vi "DCSMBReadXTemplateJK2.vi"(3 ";error in (no error)":errorcluster, 5 ";Type":i32, 6 ";DataIn 2":string) -> (0 "error IO":errorcluster, 1 "Time Stamp":timestamp, 2 ";DataIn":string)   [LabVIEW 2017]
uses:
  <vilib>/variable/detnetvar/DSV init parameters.ctl
  <vilib>/variable/detnetvar/Network provider/lvedc.dll
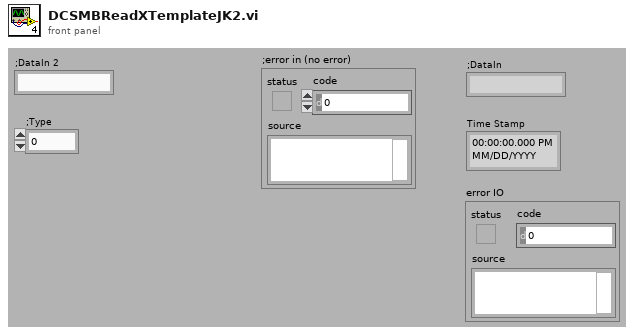
[diagram p1: front panel]
types:
  T1 = typedef "DSV init parameters.ctl" = cluster{"refIndex in":i32, "MAC Address":string, "NodeId":string, "SMB block Offset (us)":i32, "Max Variable Length":i32, "Sub Items":i32, "Item Size (bytes)":u16, "Index":i32, "SMB item Data Offset (bytes)":i32, "Timing Source Name":string, "Node is owner?":bool, "Num Items":i32, "Start Slot (us) ":i32, "GUID":string, "Reserved":string, "Cycle time (us)":i32, "Master?":bool, "Max Overall\n Message Length ":i32, "Version Count":u32, "SMB Start Times (other nodes)":i32[], "Network Speed":enum16{"100 MBit", "1 GBit"}, "SMB Variable":bool}
  T2 = typedef "DCTerminalAccessData.ctl" = cluster{"Dif":i32, "Len":i32, "User data":u32}
  T3 = typedef "DCTerminalRefNum.ctl" = cluster{"ID":i32, "GUID":dbl, "Type":enum16{"Terminal"}}
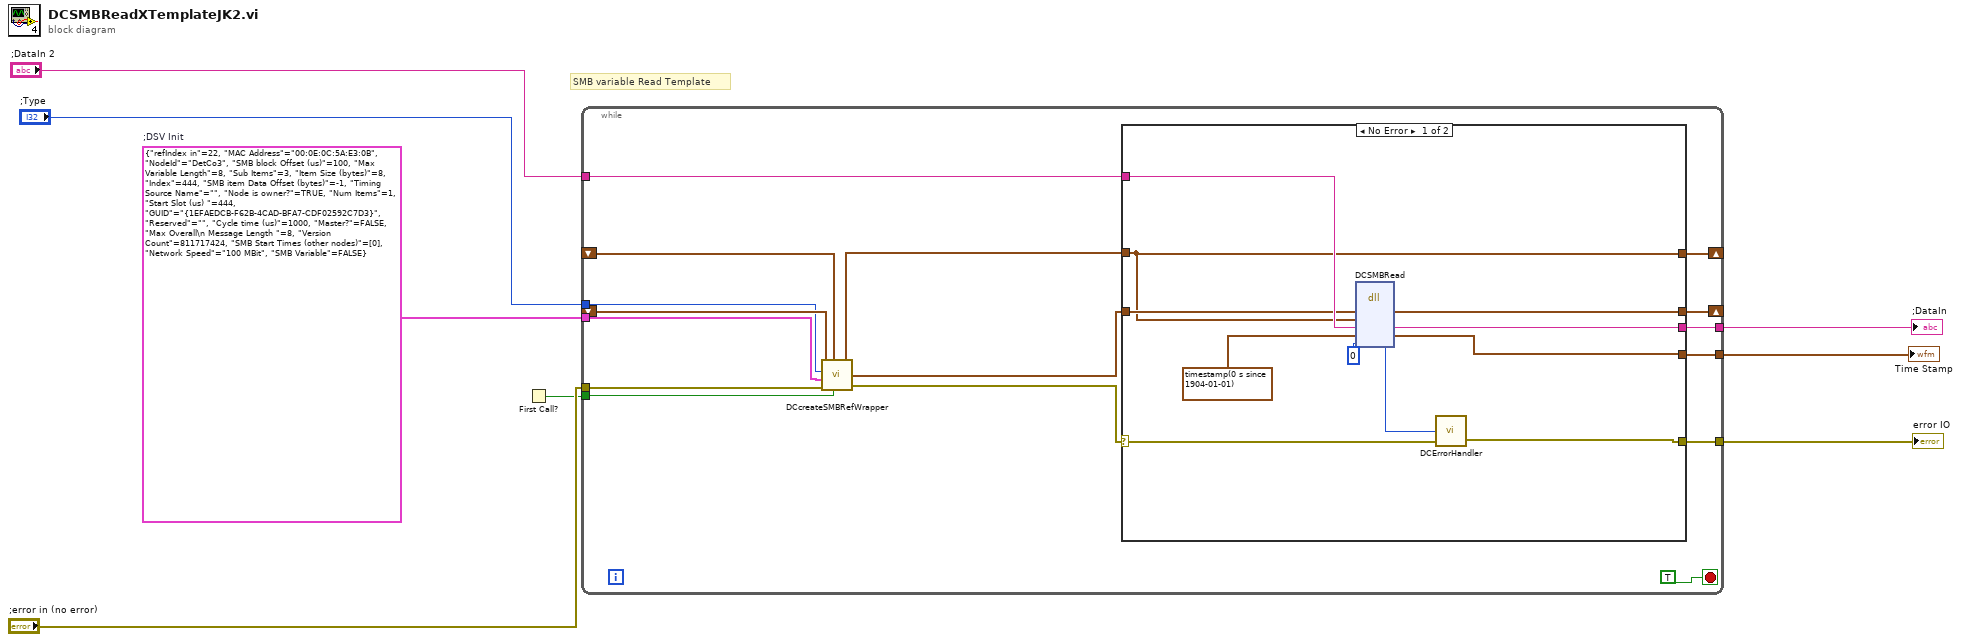
[diagram p0: block diagram]
diagram:
  w1 = T1 {"refIndex in"=22, "MAC Address"="00:0E:0C:5A:E3:0B", "NodeId"="DetCo3", "SMB block Offset (us)"=100, "Max Variable Length"=8, "Sub Items"=3, "Item Size (bytes)"=8, "Index"=444, "SMB item Data Offset (bytes)"=-1, "Timing Source Name"="", "Node is owner?"=TRUE, "Num Items"=1, "Start Slot (us) "=444, "GUID"="{1EFAEDCB-F62B-4CAD-BFA7-CDF02592C7D3}", "Reserved"="", "Cycle time (us)"=1000, "Master?"=FALSE, "Max Overall\n Message Length "=8, "Version Count"=811717424, "SMB Start Times (other nodes)"=[0], "Network Speed"=enum."100 MBit", "SMB Variable"=FALSE}  # ;DSV Init
  # "SMB variable Read Template"
  n1 = First Call?() -> (First Call?: T/F=w7:bool)
  n2 = while {
    tunnel: [w24] -> w6
    tunnel: ";error in (no error)" -> [w17]
    tunnel: ";DataIn 2" -> [w23]
    tunnel: [w22] -> w5
    shift-right: [w20] -> _
    shift-left: _ -> [w18]
    tunnel: w7 -> [w13]
    tunnel: w1 -> [w15]
    tunnel: [w14] -> w2
    tunnel: ";Type" -> [w12]
    shift-right: [w9] -> _
    shift-left: _ -> [w11]
    stop <- TRUE stop-if-true
    n3 = call <vilib>:"DCcreateSMBRefWrapper.vi"("SMB Terminal RefNum (out)"=w18, ";Terminal Data 2"=w11, ";Type"=w12, ";Init"=w15, "First Call?: T/F"=w13, ";error in (no error)"=w17) -> (";Terminal Data"=w10:T2, "SMB Terminal RefNum (out) 2"=w21:T3, "Error (out)"=w16:errorcluster)
    n4 = case shown="No Error" w16 {
      selector: w16 -> [w30 w38]
      tunnel: [w28 w38] -> w24
      tunnel: [w35 w39] -> w20
      tunnel: w10 -> [w27 w36]
      tunnel: w23 -> [w34 w37]
      tunnel: w21 -> [w33 w39]
      tunnel: [w32 w37] -> w22
      tunnel: [w25 _] -> w14
      tunnel: [w27 w36] -> w9
      frame No Error {
        n5 = dll-call lib="e:/penguin/lvdist/win32/export/17.0/17.0.0f0/dist/vi.lib/variable/detnetvar/Network provider/lvedc.dll" fn="DCSMBRead"("SMB Terminal RefNum (out) 2"=w33, ";Terminal Data"=w27, ";DataIn 2"=w34, "Time Stamp"=timestamp(0 s since 1904-01-01), "status"=0) -> ("SMB Terminal RefNum (out) 2"=w35:T3, ";DataIn 2"=w32:string, "Time Stamp"=w25:timestamp, "status"=w29:i32)  [unwired: 5 in, 2 out]
        n6 = call <vilib>:"DCErrorHandler.vi"("error in"=w30, "status"=w29) -> ("error out"=w28:errorcluster)  [unwired: 2 in]
      }
      frame Error {
      }
    }
  }
  "Time Stamp" <- w2
  "error IO" <- w6
  ";DataIn" <- w5
